vi "#11.vi"(0 "System no.":i32=1 min=1 max=4 step=1, 5 "error in":errorcluster) -> (19 "error out":errorcluster)   [LabVIEW 2020]
doc: "Returns the number of free memory points for profile definition (e.g. for a dynamic move) by sending the single ASCII character 11. \n\nC-887, F-206, M-8X0: Only for GCS syntax version = GCS 2.0 or higher (check with CSV?.vi. If CSV?.vi is not supported, syntax version is GCS 1.0)."
panel:
  out "Free trajectory points":i32 format="%x"
  # "Returns the number of free memory points for \ntrajectory definition (e.g. for a dynamic move) by \nsending the single ASCII character 11."
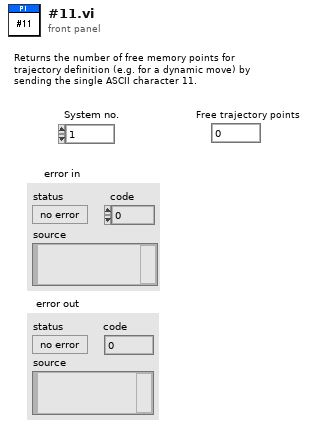
[diagram p1: front panel]
types:
  T1 = enum16{"Disable error check", "Force error check", "Use global settings"}
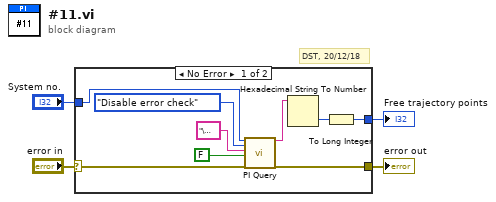
[diagram p0: block diagram]
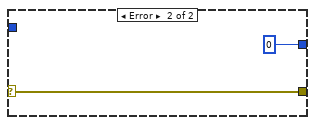
[diagram p2: hidden frame]
diagram:
  # "DST, 20/12/18"
  n1 = case shown="No Error" "error in" {
    selector: "error in" -> [w7 w15]
    tunnel: "System no." -> [w11 _]
    tunnel: [w6 0] -> w3
    tunnel: [w8 w15] -> w2
    frame No Error {
      n2 = call "PI Query.vi"("System no."=w11, "Error check settings"=T1."Disable error check", "String to send"="\u000b", "Attach termination char.?"=FALSE ("Attach Linefeed?"), "error in"=w7) -> ("String read"=w9:string, "error out"=w8:errorcluster)  [unwired: 2 in, 11 out]
      n3 = Hexadecimal String To Number(string=w9) -> (number=w10:u32)  [unwired: 3 out]
      n4 = To Long Integer(number=w10) -> (32bit integer=w6:i32)
    }
    frame Error {
    }
  }
  "error out" <- w2
  "Free trajectory points" <- w3
